vi "SVPO Convert to Even Angle Signal (1 Ch DBL WDT) with IC.vi"(0 "scaled signal [EU]":waveform(dbl)={"t0"=timestamp(0 s since 1904-01-01), "dt"=0.0, "Y"=[]}, 2 "reset? (F)":bool, 7 "speed position info":T3, 11 "initial conditions":T1={"filter prototype"={"left wing"=[], "increment"=[], "max dec"=128, "timing jitter"=enum."Interpolation", "band limiting?"=TRUE}, "interpolation filter state"={"corrected lengths"=[], "initH"=[]}, "resample state"={"signal length"=0, "time"=[], "reset state"=FALSE, "state"={"init condition"=[], "start index"=0, "channel count"=0, "condition len"=0, "position"=0.0, "time interval"=0.0, "max cond len"=0}, "offset"=0.0}} {"filter prototype"."increment" format="%.2f"; "filter prototype"."left wing" format="%.2f"}, 12 "max order":dbl=16.0) -> (4 "even-angle signal":cluster{"r0":dbl, "dr":dbl, "Y":dbl[]}={"r0"=0.0, "dr"=1.0, "Y"=[]} {"r0" format="%.2p"; "dr" format="%.2p"; "Y" format="%.2f"}, 8 "even-angle position info":T3, 15 "final conditions":T1={"filter prototype"={"left wing"=[], "increment"=[], "max dec"=128, "timing jitter"=enum."Interpolation", "band limiting?"=TRUE}, "interpolation filter state"={"corrected lengths"=[], "initH"=[]}, "resample state"={"signal length"=0, "time"=[], "reset state"=FALSE, "state"={"init condition"=[], "start index"=0, "channel count"=0, "condition len"=0, "position"=0.0, "time interval"=0.0, "max cond len"=0}, "offset"=0.0}} {"filter prototype"."increment" format="%.2f"; "filter prototype"."left wing" format="%.2f"})   [LabVIEW 2017, in "SoundVib_OrderTracking.lvlib"]
doc: "Converts an even-time-spaced scaled signal to an even-angle-spaced signal by resampling the acquired signal. The output signal is synchronous to the rotational speed with a constant number of samples per revolution. Use this VI on embedded targets that have limited computational resources. Wire data to the <B>scaled signal [EU]</B> input to determine the polymorphic instance to use or manually select the instance."
uses:
  <vilib>/addons/Sound and Vibration/Order Analysis/Resample Order Tracking/SoundVib_OrderTracking.lvlib
  <vilib>/addons/Sound and Vibration/Order Analysis/Misc/OAT Position Info.ctl
  <vilib>/addons/_NISVFA/_Shared subVIs/Controls/svc_Convert to Even Angle State.ctl
  <vilib>/addons/_NISVFA/_Shared subVIs/Controls/OAT Resample Filter Prototype.ctl
  <vilib>/addons/Sound and Vibration/Order Analysis/Resample Order Tracking/SubVIs/sv_Convert to Even Angle Signal (Generic) with IC.vi
  <vilib>/addons/Sound and Vibration/Order Analysis/Adv Resampling/oa_CIC Interpolation Filter with IC.vi
  <vilib>/addons/Sound and Vibration/Order Analysis/Adv Resampling/sv_Resample (Const to Variable, DBL Array) with IC.vi
  <vilib>/addons/Sound and Vibration/Order Analysis/Adv Resampling/sv_Resample Filter Prototype Design.vi
  <vilib>/addons/Sound and Vibration/Order Analysis/Adv Resampling/oa_Adjust Resample State Info.vi
  <vilib>/addons/Sound and Vibration/Order Analysis/Adv Resampling/OAT LP Kaiser Window Design.vi
  <vilib>/addons/Sound and Vibration/Order Analysis/Resample Order Tracking/SubVIs/oa_CIC Filter Length.vi
  <vilib>/addons/Sound and Vibration/Order Analysis/Adv Resampling/sv_Get Actual Max Order.vi
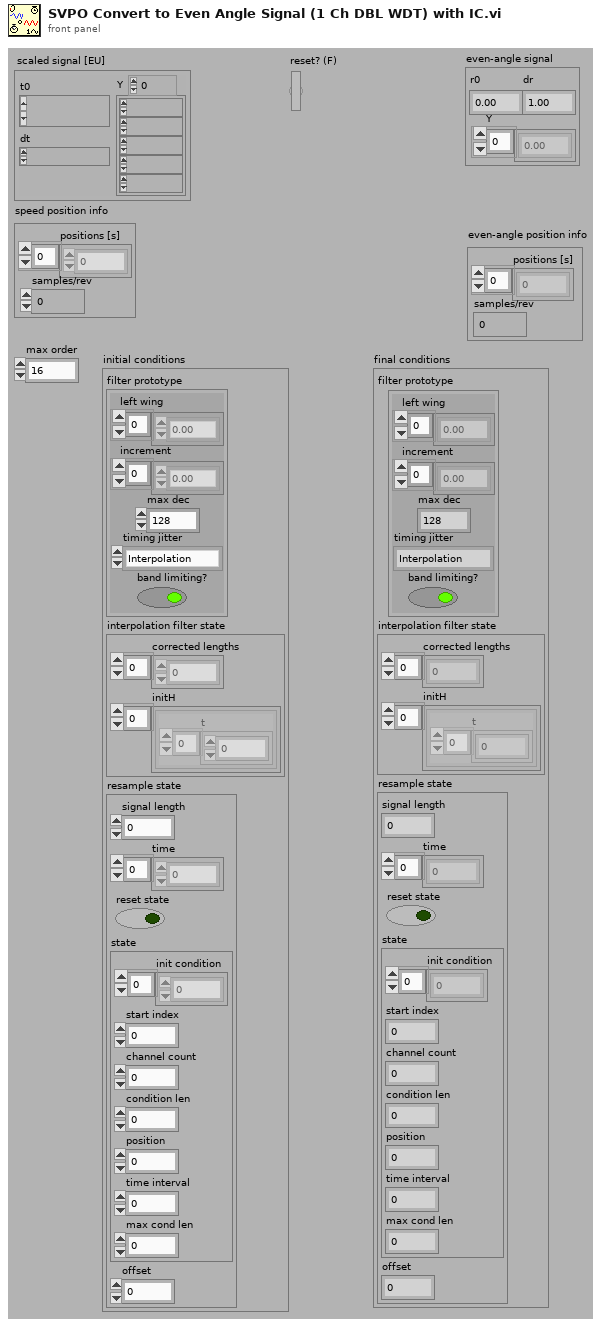
[diagram p1: front panel]
types:
  T1 = typedef "svc_Convert to Even Angle State.ctl" = cluster{"filter prototype":T2, "interpolation filter state":cluster{"corrected lengths":i32[], "initH":cluster{"t":dbl[]}[]}, "resample state":cluster{"signal length":u64, "time":dbl[], "reset state":bool, "state":cluster{"init condition":dbl[], "start index":i32, "channel count":i32, "condition len":i32, "position":dbl, "time interval":dbl, "max cond len":i32}, "offset":dbl}}
  T2 = typedef "OAT Resample Filter Prototype.ctl" = cluster{"left wing":dbl[], "increment":dbl[], "max dec":i32, "timing jitter":enum32{"Interpolation", "Rounding"}, "band limiting?":bool}
  T3 = typedef "OAT Position Info.ctl" = cluster{"positions [s]":dbl[], "samples/rev":dbl}
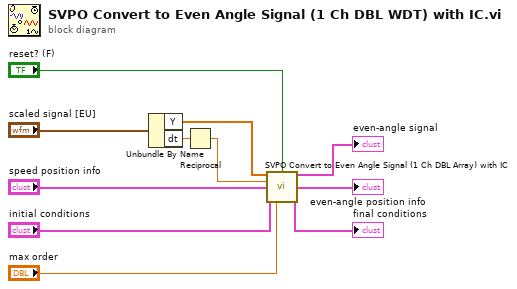
[diagram p0: block diagram]
diagram:
  n1 = Unbundle By Name("scaled signal [EU]") -> ("Y"=w10:dbl[], "dt"=w1:dbl)
  n2 = Reciprocal(x=w1) -> (1/x=w7:dbl)
  n3 = call <vilib>:"SVPO Convert to Even Angle Signal (1 Ch DBL Array) with IC.vi"("scaled signal [EU]"=w10, "reset? (F)"="reset? (F)", "sampling rate [Hz]"=w7, "speed position info"="speed position info", "initial conditions"="initial conditions", "max order"="max order") -> ("even-angle signal"=→"even-angle signal":cluster{"r0":dbl, "dr":dbl, "Y":dbl[]}, "even-angle position info"=→"even-angle position info":T3, "final conditions"=→"final conditions":T1)  [unwired: 7 in]
